vi "Init.vi"(8 "error in (no error)":errorcluster, 11 "Monkey in":refnum<class "Monkey.lvclass">) -> (0 "error out":errorcluster, 3 "Monkey out":refnum<class "Monkey.lvclass">)   [LabVIEW 2020, in "Monkey.lvlib" / "Monkey.lvclass"]
uses:
  Monkey.lvclass
  Monkey Consumer Case Selector.ctl
  Father of all uServices/Father of all uServices/Father of all uServices.lvclass
  TALOS.lvlib
  C:/Users/marco/Documents/GitHub_Lab/TALOS/talos/Father of all uServices/Father of all uServices/Father of all uServices.lvclass
  C:/Users/marco/Documents/GitHub_Lab/TALOS/talos/Ancestor/Ancestor/Ancestor.lvclass
  C:/Users/marco/Documents/GitHub_Lab/TALOS/builds/Actor Framework PPL/Actor Framework.lvlibp/1abvi3w/vi.lib/ActorFramework/Actor/Actor.lvclass
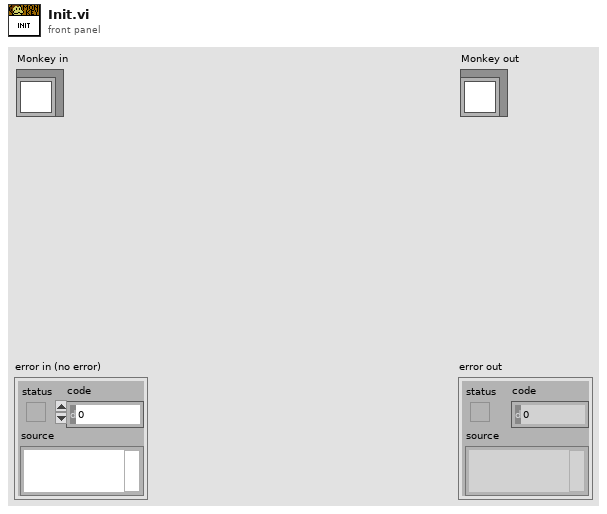
[diagram p1: front panel]
types:
  T1 = typedef "Monkey.lvlib/Monkey.lvclass/Monkey Consumer Case Selector.ctl" = enum16{"Init", "Update GUI", "New schedule", "Check Script", "Submit Script", "Banana arrived", "Optimiser - evaluate RUN", "Optimiser - update RUN", "Quality Check", "What to do next", "Update Crit Lvl", "Skip Run", "Stop Schedule", "Skip schedule"}
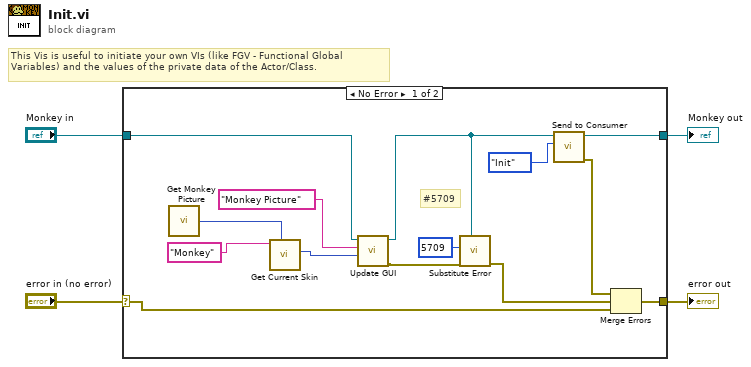
[diagram p0: block diagram]
diagram:
  # "This Vis is useful to initiate your own VIs (like FGV - Functional Global Variables) and the values of the private data of the Actor/Class."
  n1 = case shown="No Error" "error in (no error)" {
    selector: "error in (no error)" -> [w10 w19]
    tunnel: "Monkey in" -> [w5 w20]
    tunnel: [w11 w20] -> w4
    tunnel: [w14 w19] -> w3
    frame No Error {
      # "#5709"
      n2 = call "Get Monkey Picture.vi"() -> ("Monkey"=w6:picture)
      n3 = call "Get Current Skin.vi"("default"=w6, "Object"="Monkey") -> ("Picture with skin"=w7:picture)  [unwired: 4 in, 2 out]
      n4 = call "Update GUI.vi"("Data"=w7, "GUI Item Name"="Monkey Picture", "uService Template in"=w5) -> ("error out"=w17:errorcluster, "uService Template out"=w12:refnum<class "Monkey.lvclass">)  [unwired: 7 in]
      n5 = call "Substitute Error.vi"("LabVIEW Object"=w12, "error in (no error)"=w17, "Error Code"=5709) -> ("error out"=w16:errorcluster)  [unwired: 8 in]
      n6 = call "Send to Consumer.vi"("Case ID"=Monkey_Consumer_Case_Selector."Init" ("Monkey Consumer Case Selector"), "uService Template in"=w12) -> ("error out"=w15:errorcluster, "uService Template out"=w11:refnum<class "Monkey.lvclass">)  [unwired: 8 in]
      n7 = Merge Errors(w15, w16, w10) -> (w14:errorcluster)
    }
    frame Error {
    }
  }
  "error out" <- w3
  "Monkey out" <- w4
